vi "file header.vi"(8 "error in (no error)":errorcluster, 11 "Log File in":refnum<class "CCS_Log File.lvclass">) -> (0 "error out":errorcluster, 3 "Log File out":refnum<class "CCS_Log File.lvclass">)   [LabVIEW 2018, in "CCS_Log File.lvclass"]
uses:
  CCS_Log File.lvclass
  CCS_Log File.lvclass/CCS_Log File.ctl
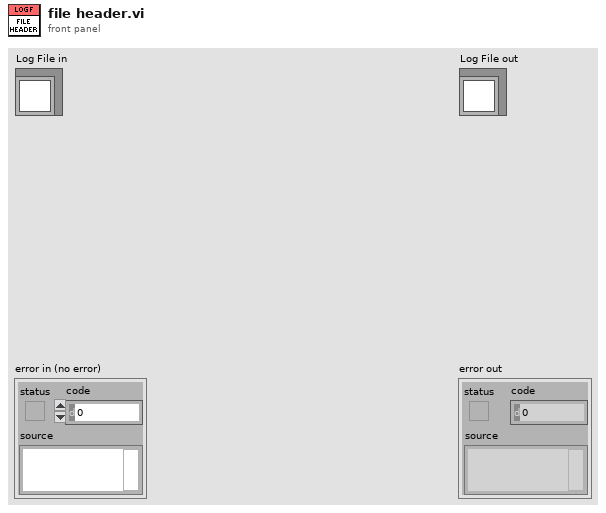
[diagram p1: front panel]
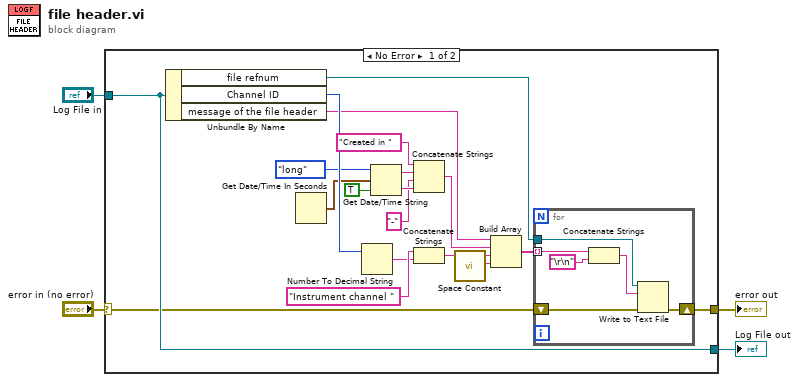
[diagram p0: block diagram]
diagram:
  n1 = case shown="No Error" "error in (no error)" {
    selector: "error in (no error)" -> [w21 w31]
    tunnel: [w20 w31] -> w3
    tunnel: [w23 w30] -> w1
    tunnel: "Log File in" -> [w23 w30]
    frame No Error {
      n2 = Unbundle By Name(w23) -> ("file refnum"=w22:refnum<file>, "Channel ID"=w16:u8, "message of the file header"=w5:string)
      n3 = Get Date/Time In Seconds() -> (seconds since 1Jan1904=w15:timestamp)
      n4 = Number To Decimal String(number=w16) -> (decimal integer string=w17:string)  [unwired: 1 in]
      n5 = Get Date/Time String(date format (0)=enum16{"short", "long", "abbreviated"}."long", seconds (now)=w15, want seconds? (F)=TRUE) -> (date string=w14:string, time string=w13:string)
      n6 = Concatenate Strings("Created in ", w14, "-" ("string"), w13) -> (w7:string)
      n7 = Concatenate Strings("Instrument channel ", w17) -> (w6:string)
      n8 = call <vilib>:"Space Constant.vi"() -> ("String"=w8:string)
      n9 = Build Array(w5, w7, w6, w8) -> (w19:string[])
      n10 = for {
        tunnel: w22 -> [w29]
        shift-right: [w27] -> w20
        shift-left: w21 -> [w28]
        tunnel: w19 -> [w26] mode=indexing
        n11 = Concatenate Strings(w26, "\r\n") -> (w24:string)
        n12 = Write to Text File(file (use dialog)=w29, text=w24, error in=w28) -> (error out=w27:errorcluster)  [unwired: 1 in, 2 out]
      }
    }
    frame Error {
    }
  }
  "error out" <- w3
  "Log File out" <- w1
